vi "json Parse Variant - string path.vi"(8 "error in (no error)":errorcluster, 9 "default":variant, 10 "path":string, 11 "JSON Document in":refnum<class "JSON Document.lvclass">) -> (0 "error out":errorcluster, 1 "defaulted?":bool, 2 "value":variant, 3 "JSON Document out":refnum<class "JSON Document.lvclass">)   [LabVIEW 2015, in "JSON Document.lvclass"]
uses:
  JSON Document.lvclass
  json Parse String - string path.vi
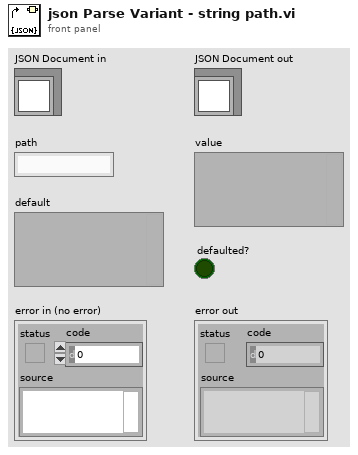
[diagram p1: front panel]
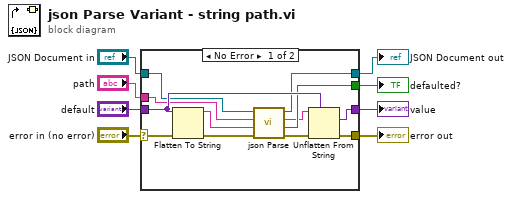
[diagram p0: block diagram]
diagram:
  n1 = case shown="No Error" "error in (no error)" {
    selector: "error in (no error)" -> [w18 w23]
    tunnel: [w17 w23] -> w7
    tunnel: [w11 w22] -> w5
    tunnel: "JSON Document in" -> [w13 w22]
    tunnel: "default" -> [w20 w21]
    tunnel: "path" -> [w19 _]
    tunnel: [w16 w21] -> w2
    tunnel: [w12 _] -> w1
    frame No Error {
      n2 = Flatten To String(anything=w20, error in (no error)=w18) -> (data string=w10:string, error out=w15:errorcluster)  [unwired: 2 in, 1 out]
      n3 = call-poly "json Parse.vi"("error in (no error)"=w15, "default"=w10, "path"=w19, "JSON Document in"=w13) -> ("error out"=w14:errorcluster, "defaulted?"=w12:bool, "value"=w9:string, "JSON Document out"=w11:refnum<class "JSON Document.lvclass">)  [unwired: 4 in]
      n4 = Unflatten From String(type=w20, binary string=w9, error in (no error)=w14) -> (value=w16:variant, error out=w17:errorcluster)  [unwired: 2 in, 1 out]
    }
    frame Error {
    }
  }
  "error out" <- w7
  "JSON Document out" <- w5
  "value" <- w2
  "defaulted?" <- w1
